vi "oa_Number of Blocks and Output Initialized Array.vi"(6 "block size":i32=1024, 8 "index":i32, 9 "dr":dbl=1.0, 10 "trigger period [rev]":dbl=1.0, 11 "even angle signal":dbl[](array[numeric])) -> (0 "initialized array":dbl[](array[numeric]), 3 "number of blocks":i32)   [LabVIEW 2017, in "SoundVib_OAUtility.lvlib"]
uses:
  <vilib>/addons/Sound and Vibration/Order Analysis/Utility/SoundVib_OAUtility.lvlib
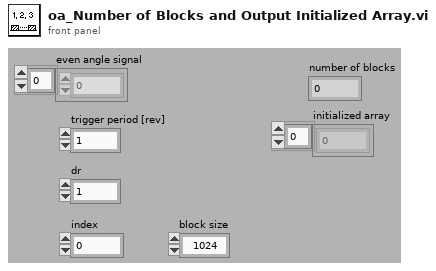
[diagram p1: front panel]
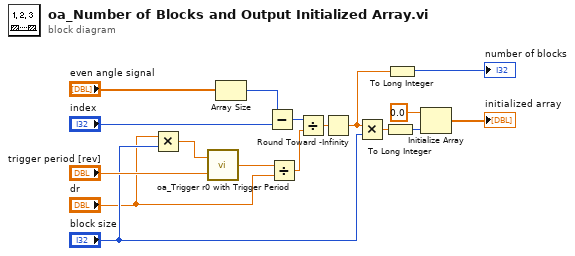
[diagram p0: block diagram]
diagram:
  n1 = Multiply(x="dr", y="block size") -> (x*y=w10:dbl)
  n2 = call <vilib>:"oa_Trigger r0 with Trigger Period.vi"("trigger period [rev]"="trigger period [rev]", "r0"=w10) -> ("triggered r0"=w9:dbl)
  n3 = Array Size(array="even angle signal") -> (size(s)=w17:i32)
  n4 = Subtract(x=w17, y="index") -> (x-y=w16:i32)
  n5 = Divide(x=w9, y="dr") -> (x/y=w11:dbl)
  n6 = Divide(x=w16, y=w11) -> (x/y=w12:dbl)
  n7 = Round Toward -Infinity(1:w12) -> (0:w1:dbl)
  n8 = Multiply(x=w1, y="block size") -> (x*y=w14:dbl)
  n9 = To Long Integer(number=w14) -> (32bit integer=w15:i32)
  n10 = To Long Integer(number=w1) -> (32bit integer=→"number of blocks":i32)
  n11 = Initialize Array(0.0 ("element"), w15) -> (→"initialized array":dbl[])
